vi "三段比较器（STR[]).vi"(1 "低":string, 2 "输入字符串":string[](array[string]), 3 "高":string) -> (0 "Range":enum16{"超低", "适中", "超高"}[](array[ring]))   [LabVIEW 2011]
doc: "功能：\n\n返回一个枚举，表明输入数的范围，用于三段比较。\n\n\nCSXCS_366创建。"
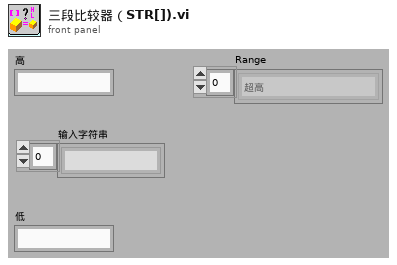
[diagram p1: front panel]
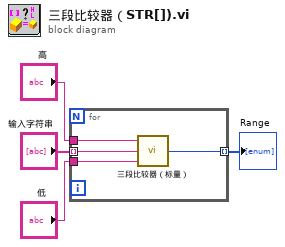
[diagram p0: block diagram]
diagram:
  n1 = for {
    tunnel: "高" -> [w8]
    tunnel: "输入字符串" -> [w7] mode=indexing
    tunnel: "低" -> [w6]
    tunnel: [w5] -> w1 mode=indexing
    n2 = call-poly "三段比较器（标量）.vi"("低"=w6, "输入字符串"=w7, "高"=w8) -> ("Range"=w5:enum16{"超低", "适中", "超高"})
  }
  "Range" <- w1
